vi "Test DQMH_byOOPRef API.vi"() -> ()   [LabVIEW 2021]
doc: "DQMH_byOOPRef API Tester."
uses:
  DQMH_byOOPRef.lvlib
  <vilib>/Utility/error.llb/DialogType.ctl
panel:
  in  "Second Event String Update":bool
  in  "Event String Update":bool
  out "last error":errorcluster
  in  "Show Diagram on Init":bool
  in  "Run as Singleton?":bool
  in  "Show Block Diagram":bool
  in  "Refresh Modules":bool
  out "Active Modules":string[](array[string])
  in  "Stop Module":bool
  in  "Select Module":i32(ring)=-1 caption="Select Module\nTo send Request to" items=["All"=-1]
  in  "Run New Module":bool
  in  "Hide Module Panel":bool
  in  "Show Module Panel":bool
  out "Status":string
  # "This VI tests the API for the Module."
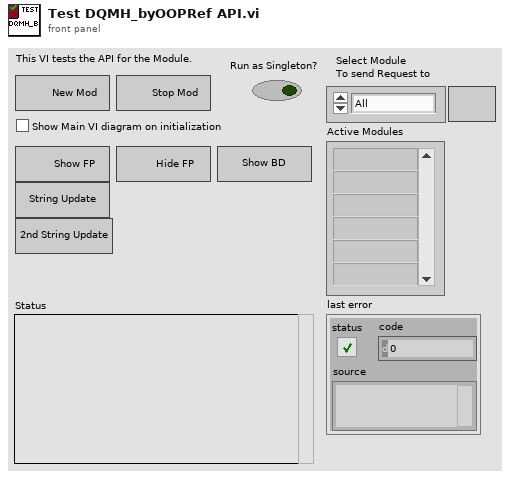
[diagram p1: front panel]
types:
  T1 = typedef "DQMH_byOOPRef.lvlib/Broadcast Events--cluster.ctl" = cluster{"Module Did Init":refnum<user-event>, "Status Updated":refnum<user-event>, "Error Reported":refnum<user-event>, "Module Did Stop":refnum<user-event>, "Update Module Execution Status":refnum<user-event>}
  T2 = typedef "DialogType.ctl" = u16
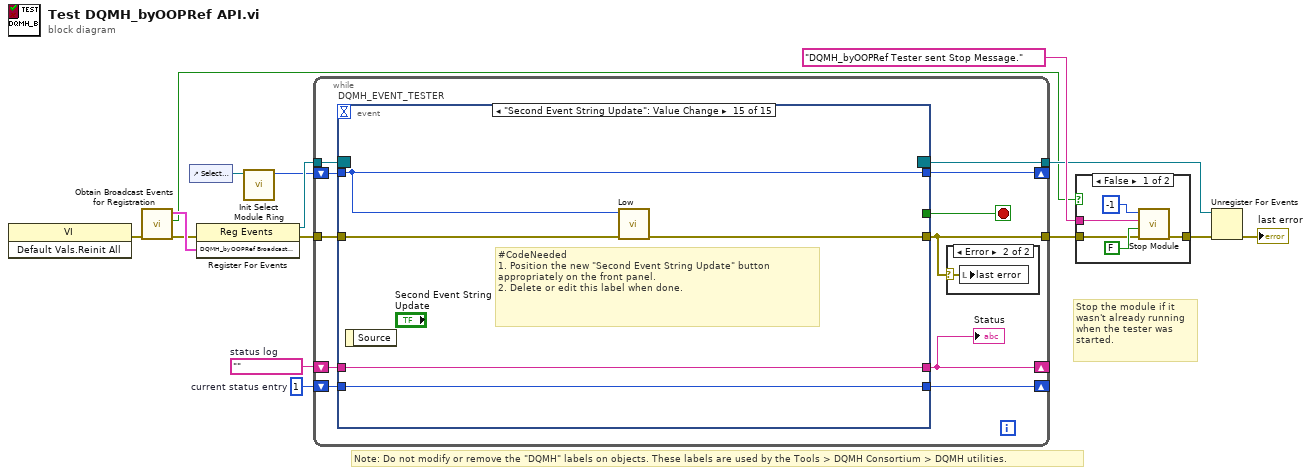
[diagram p0: block diagram]
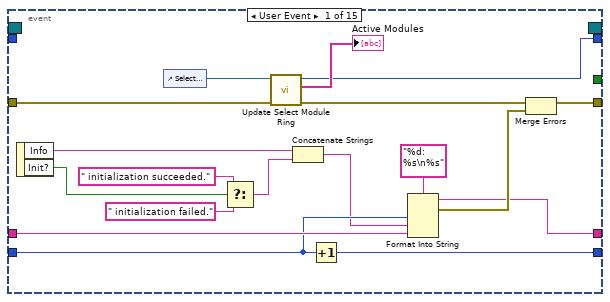
[diagram p4: hidden frame]
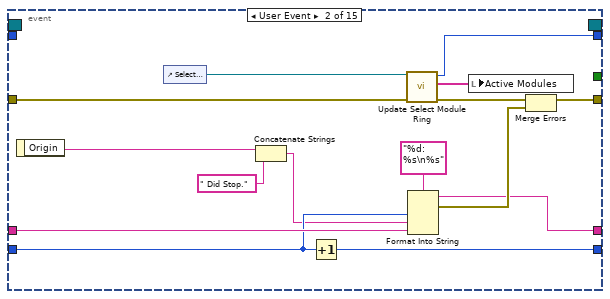
[diagram p5: hidden frame]
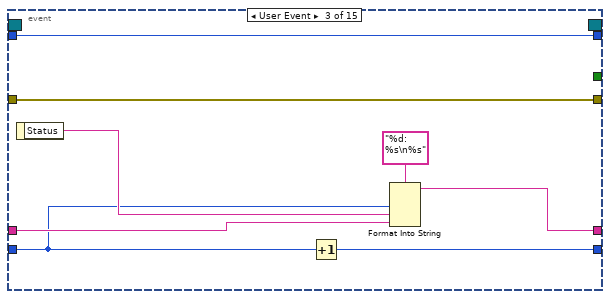
[diagram p6: hidden frame]
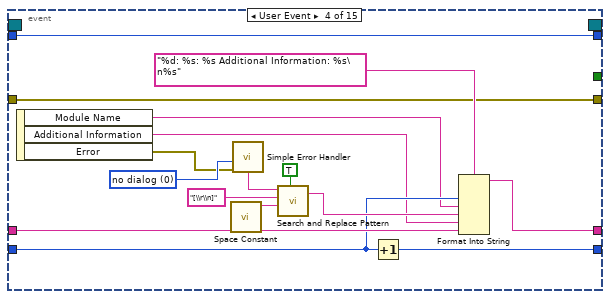
[diagram p7: hidden frame]
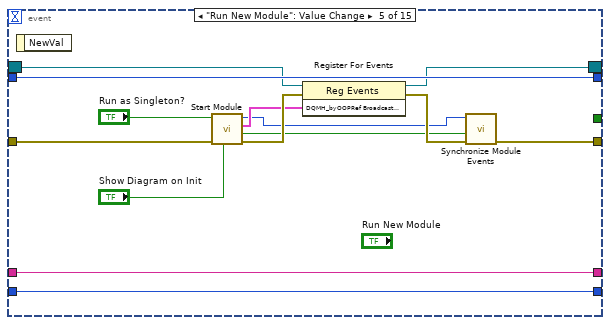
[diagram p8: hidden frame]
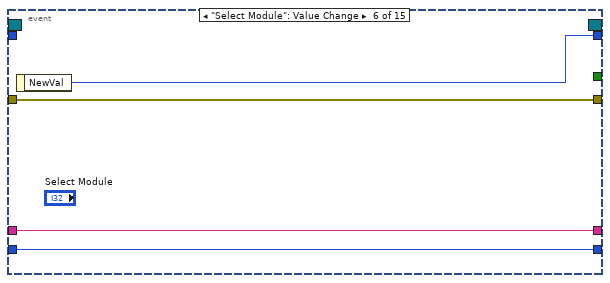
[diagram p9: hidden frame]
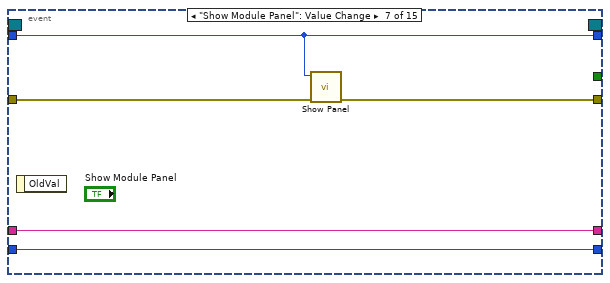
[diagram p10: hidden frame]
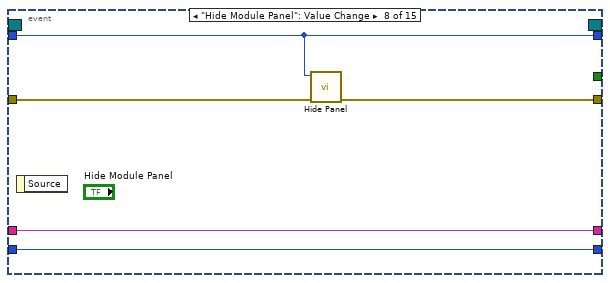
[diagram p11: hidden frame]
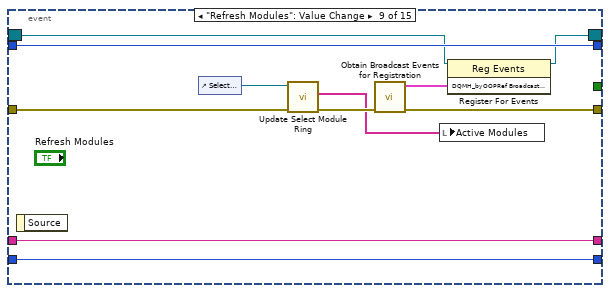
[diagram p12: hidden frame]
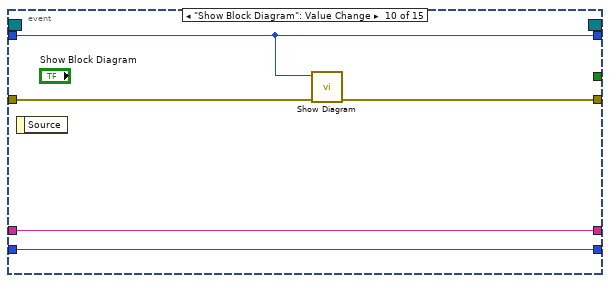
[diagram p13: hidden frame]
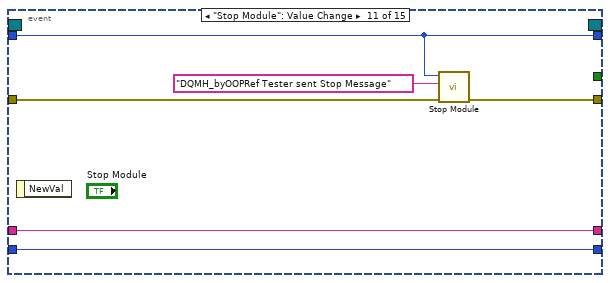
[diagram p14: hidden frame]
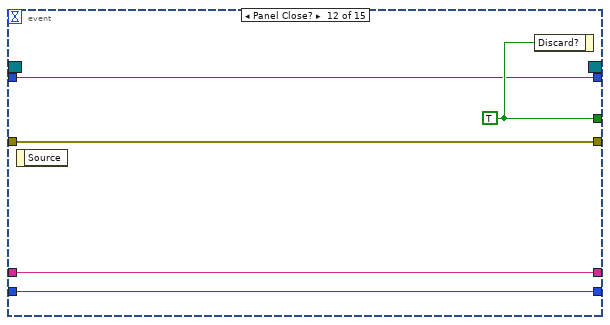
[diagram p15: hidden frame]
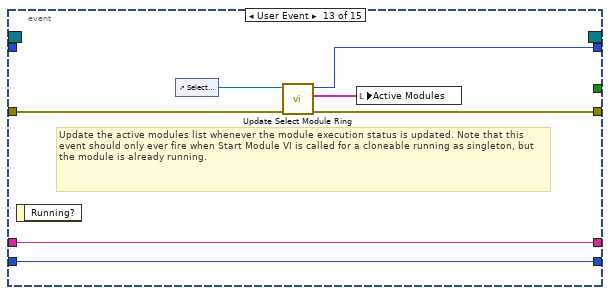
[diagram p16: hidden frame]
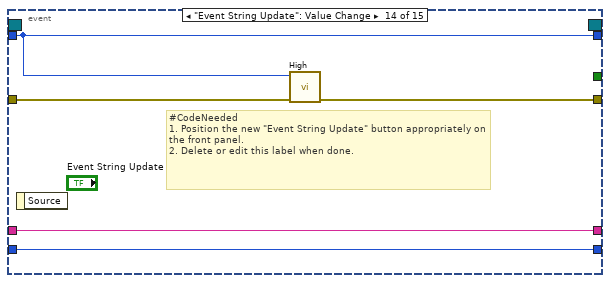
[diagram p17: hidden frame]
diagram:
  w12 = 1  # current status entry
  w13 = ""  # status log
  # "Stop the module if it wasn't already running when the tester was started."
  # "Note: Do not modify or remove the \"DQMH\" labels on objects. These labels are used by the Tools > DQMH Consortium > DQMH utilities."
  n1 = invoke class="VI" method="Default Vals.Reinit All"() -> (error out=w5:errorcluster)  [unwired: 3 in, 2 out]
  n2 = call "Obtain Broadcast Events for Registration.vi"("error in"=w5) -> ("error out"=w4:errorcluster, "Already running?"=w3:bool, "DQMH_byOOPRef Broadcast Events"=w9:T1)  [unwired: 8 in]
  n3 = control-ref of="Select Module"() -> (w10:refnum<vi>)
  n4 = register-events(error in=w4, w9) -> (reference out=w15:refnum<event-registration>, error out=w8:errorcluster)  [unwired: 1 in]
  n5 = call "Init Select Module Ring.vi"("Select Module Ring Ref"=w10) -> ("Value for All Modules"=w11:i32)  [unwired: 8 in, 2 out]
  n6 = while {
    tunnel: w15 -> [w26]
    tunnel: [w17] -> w2
    tunnel: w8 -> [w25]
    shift-right: [w21] -> _
    shift-left: w13 -> [w23]
    shift-right: [w22] -> _
    shift-left: w12 -> [w24]
    shift-right: [w19] -> _
    shift-left: w11 -> [w20]
    tunnel: [w18] -> w6
    stop <- w16 stop-if-true
    n7 = event "DQMH_EVENT_TESTER" shown="[14] \"Second Event String Update\": Value Change" {
      selector: w26 -> [_ _ _ _ w92 _ _ _ w118 _ _ _ _ _ _]
      dyn-events: [_ _ _ _ w91 _ _ _ w117 _ _ _ _ _ _] -> w18
      timeout: _ -> [_ _ _ _ _ _ _ _ _ _ _ _ _ _ _]
      tunnel: [_ _ _ _ _ _ _ _ _ _ _ w139 _ _ _] -> w16
      tunnel: [w35 w52 w68 w72 w90 w102 w106 w111 w114 w125 w130 w138 w142 w147 w152] -> w17
      tunnel: w25 -> [w37 w54 w68 w72 w93 w102 w107 w112 w119 w128 w131 w138 w143 w151 w156]
      tunnel: w24 -> [w42 w57 w61 w75 w95 w100 w104 w109 w122 w126 w133 w136 w145 w149 w154]
      tunnel: w23 -> [w43 w58 w64 w76 w96 w101 w105 w110 w123 w127 w134 w137 w146 w150 w155]
      tunnel: [w40 w55 w65 w74 w96 w101 w105 w110 w123 w127 w134 w137 w146 w150 w155] -> w21
      tunnel: [w41 w56 w67 w73 w95 w100 w104 w109 w122 w126 w133 w136 w145 w149 w154] -> w22
      tunnel: w20 -> [_ _ w62 w84 w94 _ w103 w108 w121 w124 w132 w135 _ w148 w153]
      tunnel: [w32 w49 w62 w84 w94 w99 w103 w108 w121 w124 w132 w135 w141 w148 w153] -> w19
      event User Event {
        n8 = event-data() -> ("Info"=w39:string, "Init?"=w29:bool)  [unwired: 1 in]
        n9 = control-ref of="Select Module"() -> (w34:refnum<vi>)
        n10 = Select(t=" initialization succeeded.", s=w29, f=" initialization failed.") -> (s? t:f=w28:string)
        n11 = call "Update Select Module Ring.vi"("error in"=w37, "Select Module Ring Ref"=w34) -> ("error out"=w36:errorcluster, "Active Modules (Array)"=→"Active Modules":string[], "New Module Ring Value"=w32:i32)  [unwired: 7 in]
        n12 = Concatenate Strings(w39, w28) -> (w38:string)
        n13 = Increment(x=w42) -> (x+1=w41:i32)
        n14 = Format Into String(format string="%d: %s\n%s", w42, w38, w43) -> (resulting string=w40:string, error out=w45:errorcluster)  [unwired: 2 in]
        n15 = Merge Errors(w36, w45) -> (w35:errorcluster)
      }
      event User Event {
        n16 = event-data() -> ("Origin"=w47:string)  [unwired: 1 in]
        n17 = control-ref of="Select Module"() -> (w51:refnum<vi>)
        n18 = Concatenate Strings(w47, " Did Stop.") -> (w46:string)
        n19 = Increment(x=w57) -> (x+1=w56:i32)
        n20 = call "Update Select Module Ring.vi"("error in"=w54, "Select Module Ring Ref"=w51) -> ("error out"=w53:errorcluster, "Active Modules (Array)"=w50:string[], "New Module Ring Value"=w49:i32)  [unwired: 7 in]
        n21 = Format Into String(format string="%d: %s\n%s", w57, w46, w58) -> (resulting string=w55:string, error out=w60:errorcluster)  [unwired: 2 in]
        n22 = local write "Active Modules"(w50) -> ()
        n23 = Merge Errors(w53, w60) -> (w52:errorcluster)
      }
      event User Event {
        n24 = event-data() -> ("Status"=w63:string)  [unwired: 1 in]
        n25 = Increment(x=w61) -> (x+1=w67:i32)
        n26 = Format Into String(format string="%d: %s\n%s", w61, w63, w64) -> (resulting string=w65:string)  [unwired: 2 in, 1 out]
      }
      event User Event {
        w77 = T2 0 items=["no dialog", "OK message", "continue or stop message", "OK message + warnings", "continue/stop + warnings"] ("type of dialog (OK msg:1)")
        n27 = event-data() -> ("Module Name"=w71:string, "Additional Information"=w70:string, "Error"=w69:errorcluster)  [unwired: 1 in]
        n28 = call <vilib>:"Space Constant.vi"() -> ("String"=w81:string)
        n29 = call <vilib>:"Simple Error Handler.vi"("type of dialog (OK msg:1)"=w77, "error in (no error)"=w69) -> ("message"=w78:string)  [unwired: 3 in, 4 out]
        n30 = call <vilib>:"Search and Replace Pattern.vi"("string"=w78, "regular expression (\"\")"="[\\r\\n]" ("regular expression (\"\")"), "replace string (\"\")"=w81, "replace all? (F)"=TRUE ("replace all CR/LF with spaces")) -> ("result string"=w79:string)  [unwired: 1 in, 1 out]
        n31 = Increment(x=w75) -> (x+1=w73:i32)
        n32 = Format Into String(format string="%d: %s: %s Additional Information: %s\n%s", w75, w71, w79, w70, w76) -> (resulting string=w74:string)  [unwired: 2 in, 1 out]
      }
      event "Run New Module": Value Change {
        n33 = event-data() -> ()  [unwired: 1 in, 1 out]
        n34 = call "Start Module.vi"("Show Main VI Diagram on Init (F)"="Show Diagram on Init", "error in"=w93, "Run as Singleton? (F)"="Run as Singleton?") -> ("error out"=w97:errorcluster, "Wait for Event Sync?"=w89:bool, "DQMH_byOOPRef Broadcast Events"=w88:T1, "Module ID"=w85:i32)  [unwired: 5 in]
        n35 = register-events(reference=w92, error in=w97, w88) -> (reference out=w91:refnum<event-registration>, error out=w98:errorcluster)
        n36 = call "Synchronize Module Events.vi"("error in"=w98, "Wait for Event Sync?"=w89, "Module ID in"=w85) -> ("error out"=w90:errorcluster)  [unwired: 7 in, 1 out]
      }
      event "Select Module": Value Change {
        n37 = event-data() -> ("NewVal"=w99:i32)  [unwired: 1 in]
      }
      event "Show Module Panel": Value Change {
        n38 = event-data() -> ()  [unwired: 1 in, 1 out]
        n39 = call "Show Panel.vi"("error in"=w107, "Module ID"=w103) -> ("error out"=w106:errorcluster)  [unwired: 9 in]
      }
      event "Hide Module Panel": Value Change {
        n40 = event-data() -> ()  [unwired: 1 in, 1 out]
        n41 = call "Hide Panel.vi"("error in"=w112, "Module ID"=w108) -> ("error out"=w111:errorcluster)  [unwired: 9 in]
      }
      event "Refresh Modules": Value Change {
        n42 = event-data() -> ()  [unwired: 1 in, 1 out]
        n43 = control-ref of="Select Module"() -> (w120:refnum<vi>)
        n44 = call "Update Select Module Ring.vi"("error in"=w119, "Select Module Ring Ref"=w120) -> ("error out"=w115:errorcluster, "Active Modules (Array)"=w113:string[])  [unwired: 7 in, 1 out]
        n45 = call "Obtain Broadcast Events for Registration.vi"("error in"=w115) -> ("error out"=w114:errorcluster, "DQMH_byOOPRef Broadcast Events"=w116:T1)  [unwired: 8 in, 1 out]
        n46 = local write "Active Modules"(w113) -> ()
        n47 = register-events(reference=w118, w116) -> (reference out=w117:refnum<event-registration>)  [unwired: 1 in, 1 out]
      }
      event "Show Block Diagram": Value Change {
        n48 = event-data() -> ()  [unwired: 1 in, 1 out]
        n49 = call "Show Diagram.vi"("error in"=w128, "Module ID"=w124) -> ("error out"=w125:errorcluster)  [unwired: 9 in]
      }
      event "Stop Module": Value Change {
        n50 = event-data() -> ()  [unwired: 1 in, 1 out]
        n51 = call "Stop Module.vi"("error in"=w131, "Origin"="DQMH_byOOPRef Tester sent Stop Message", "Module ID"=w132) -> ("error out"=w130:errorcluster)  [unwired: 8 in]
      }
      event Panel Close? {
        w139 = TRUE ("Discard?")
        n52 = event-data() -> ()  [unwired: 1 in, 1 out]
        n53 = event-data("Discard?"=w139) -> ()  [unwired: 1 in, 1 out]
      }
      event User Event {
        # "Update the active modules list whenever the module execution status is updated. Note that this event should only ever fire when Start Module VI is called for a cloneable running as singleton, but the module is already running."
        n54 = event-data() -> ()  [unwired: 1 in, 1 out]
        n55 = control-ref of="Select Module"() -> (w144:refnum<vi>)
        n56 = call "Update Select Module Ring.vi"("error in"=w143, "Select Module Ring Ref"=w144) -> ("error out"=w142:errorcluster, "Active Modules (Array)"=w140:string[], "New Module Ring Value"=w141:i32)  [unwired: 7 in]
        n57 = local write "Active Modules"(w140) -> ()
      }
      event "Event String Update": Value Change {
        # "#CodeNeeded\n1. Position the new \"Event String Update\" button appropriately on the front panel.\n2. Delete or edit this label when done."
        n58 = event-data() -> ()  [unwired: 1 in, 1 out]
        n59 = call "High.vi"("error in"=w151, "Module ID"=w148) -> ("error out"=w147:errorcluster)  [unwired: 8 in, 1 out]
      }
      event "Second Event String Update": Value Change {
        # "#CodeNeeded\n1. Position the new \"Second Event String Update\" button appropriately on the front panel.\n2. Delete or edit this label when done."
        n60 = event-data() -> ()  [unwired: 1 in, 1 out]
        n61 = call "Low.vi"("error in"=w156, "Module ID"=w153) -> ("error out"=w152:errorcluster)  [unwired: 9 in]
      }
    }
    "Status" <- w21
    n62 = case shown="Error" w17 {
      selector: w17 -> [_ w27]
      frame No Error {
      }
      frame Error {
        n63 = local write "last error"(w27) -> ()
      }
    }
  }
  n64 = case shown="False" w3 {
    tunnel: [w161 w162] -> w14
    tunnel: "DQMH_byOOPRef Tester sent Stop Message." ("Origin") -> [w160 _]
    tunnel: w2 -> [w157 w162]
    frame False {
      n65 = call "Stop Module.vi"("error in"=w157, "Wait for Module to stop? (F)"=FALSE ("Wait for Module to stop?"), "Origin"=w160, "Module ID"=-1 ("Stop all")) -> ("error out"=w161:errorcluster)  [unwired: 7 in]
    }
    frame True {
    }
  }
  n66 = Unregister For Events(event registration refnum=w6, error in=w14) -> (error out=→"last error":errorcluster)
